vi "Ltree array to JSON.vi"(10 "Values":string[](array[string]), 11 "Names":string[][](array[string])) -> (3 "JSON String":string)   [LabVIEW 2019, in "Userlib.lvlib"]
uses:
  Userlib.lvlib
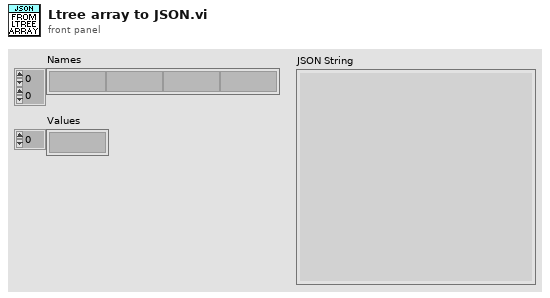
[diagram p1: front panel]
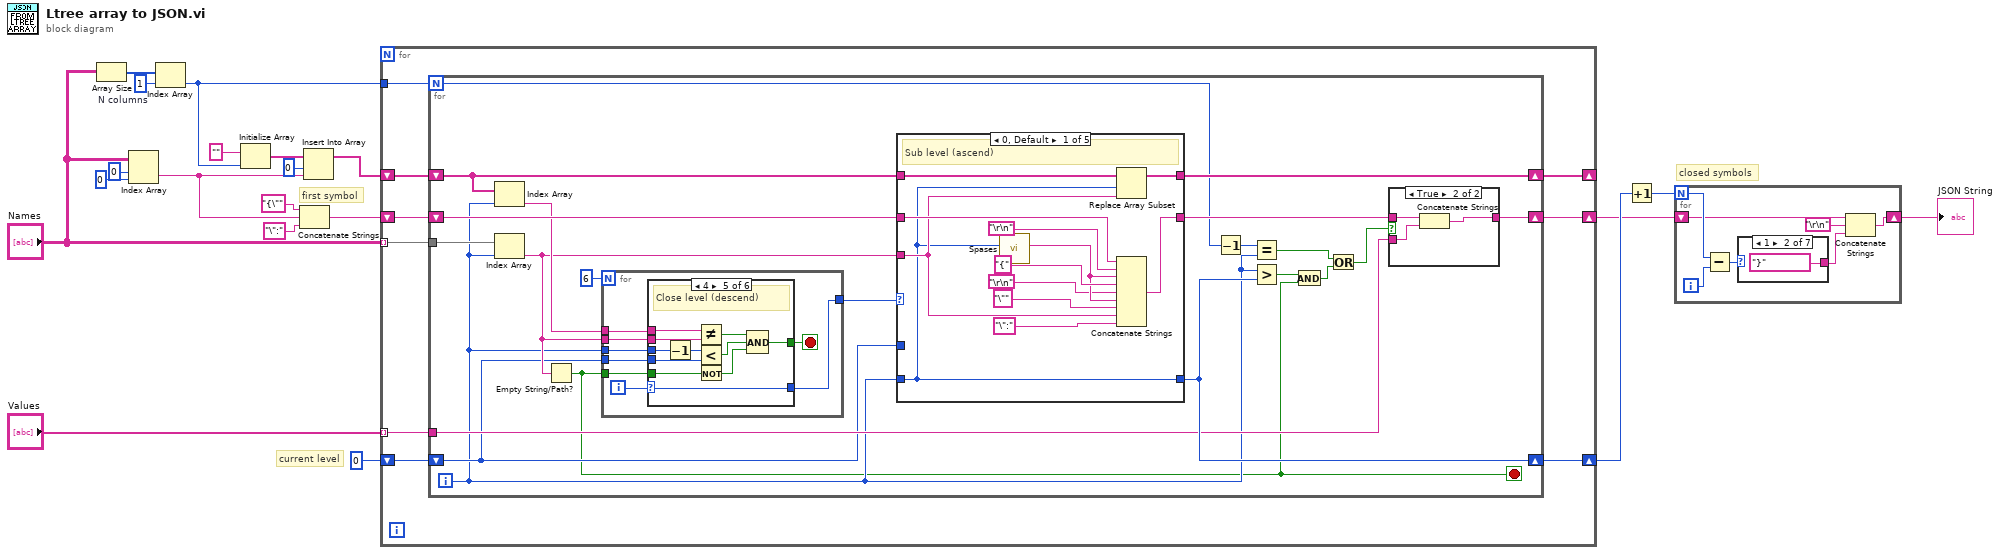
[diagram p0: block diagram]
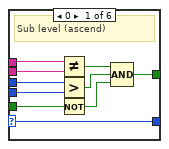
[diagram p2: hidden frame]
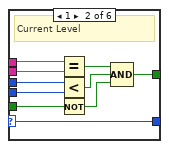
[diagram p3: hidden frame]
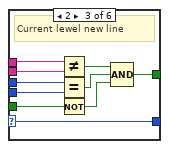
[diagram p4: hidden frame]
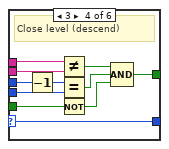
[diagram p5: hidden frame]
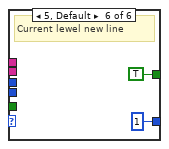
[diagram p6: hidden frame]
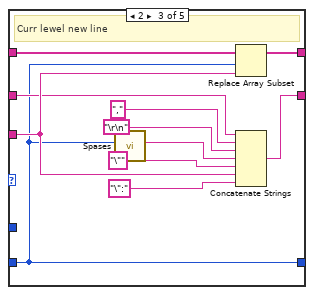
[diagram p8: hidden frame]
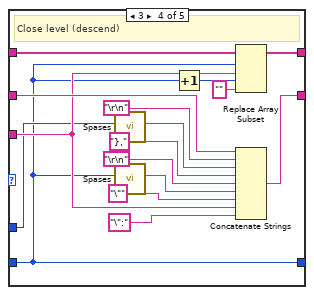
[diagram p9: hidden frame]
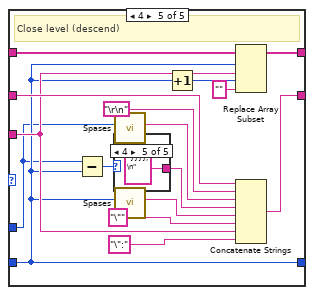
[diagram p10: hidden frame]
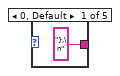
[diagram p11: hidden frame]
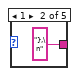
[diagram p12: hidden frame]
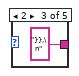
[diagram p13: hidden frame]
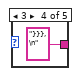
[diagram p14: hidden frame]
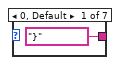
[diagram p16: hidden frame]
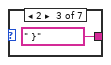
[diagram p17: hidden frame]
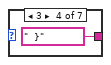
[diagram p18: hidden frame]
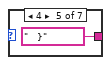
[diagram p19: hidden frame]
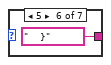
[diagram p20: hidden frame]
diagram:
  w18 = 1  # N columns
  # "closed symbols"
  # "first symbol"
  # "current level"
  n1 = Array Size(array="Names") -> (size(s)=w19:i32[])
  n2 = Index Array(array="Names", index (row)=0, index (col)=0 ("disabled index (col)")) -> (element=w10:string)
  n3 = Index Array(array=w19, index=w18) -> (element=w5:i32)
  n4 = Initialize Array("", w5) -> (w12:string[])
  n5 = Concatenate Strings("{\"", w10, "\":" ("string")) -> (w13:string)
  n6 = Insert Into Array(array=w12, index=0, new element=w10) -> (w9:string[])
  n7 = for {
    tunnel: "Names" -> [w26] mode=indexing
    shift-right: [w27] -> w7
    shift-left: w13 -> [w28]
    shift-right: [w24] -> w8
    shift-left: 0 -> [w25]
    shift-right: [w23] -> _
    shift-left: w9 -> [w29]
    tunnel: w5 -> [w22]
    tunnel: "Values" -> [w21] mode=indexing
    n8 = for {
      N: w22 -> [w34]
      tunnel: w26 -> [w47]
      shift-right: [w49] -> w23
      shift-left: w29 -> [w50]
      shift-right: [w45] -> w27
      shift-left: w28 -> [w48]
      shift-right: [w43] -> w24
      shift-left: w25 -> [w39]
      tunnel: w21 -> [w42]
      i -> [w35]
      stop <- w30 stop-if-true
      n9 = Index Array(array=w50, index=w35) -> (element=w41:string)
      n10 = Index Array(array=w47, index=w35) -> (element=w40:string)
      n11 = Empty String/Path?(string/path=w40) -> (empty?=w30:bool)
      n12 = for {
        N: 6 -> [_]
        tunnel: w41 -> [w58]
        tunnel: w40 -> [w57]
        tunnel: w39 -> [w56]
        tunnel: w30 -> [w55]
        tunnel: w35 -> [w54]
        tunnel: [w51] -> w38
        i -> [w52]
        stop <- w53 stop-if-true
        n13 = case shown="4" w52 {
          selector: w52 -> [w59 w69 w79 w89 w100 _]
          tunnel: w58 -> [w65 w75 w85 w96 w107 _]
          tunnel: w57 -> [w64 w74 w84 w95 w106 _]
          tunnel: w54 -> [w63 w73 w83 w91 w102 _]
          tunnel: w56 -> [w62 w72 w82 w94 w105 _]
          tunnel: w55 -> [w61 w71 w81 w93 w104 _]
          tunnel: [w60 w70 w80 w92 w103 TRUE] -> w53
          tunnel: [w59 w69 w79 w89 w100 1] -> w51
          frame 0 {
            # "Sub level (ascend)"
            n14 = Not Equal?(x=w65, y=w64) -> (x != y?=w68:bool)
            n15 = Greater?(x=w63, y=w62) -> (0:w67:bool)
            n16 = Not(x=w61) -> (.not. x?=w66:bool)
            n17 = Compound Arithmetic op=AND(w68, w67, w66) -> (w60:bool)
          }
          frame 1 {
            # "Current Level"
            n18 = Equal?(x=w75, y=w74) -> (x = y?=w78:bool)
            n19 = Less?(x=w73, y=w72) -> (x < y?=w77:bool)
            n20 = Not(x=w71) -> (.not. x?=w76:bool)
            n21 = Compound Arithmetic op=AND(w78, w77, w76) -> (w70:bool)
          }
          frame 2 {
            # "Current lewel new line"
            n22 = Not Equal?(x=w85, y=w84) -> (x != y?=w88:bool)
            n23 = Equal?(x=w83, y=w82) -> (x = y?=w87:bool)
            n24 = Not(x=w81) -> (.not. x?=w86:bool)
            n25 = Compound Arithmetic op=AND(w88, w87, w86) -> (w80:bool)
          }
          frame 3 {
            # "Close level (descend)"
            n26 = Decrement(x=w91) -> (x-1=w90:i32)
            n27 = Not Equal?(x=w96, y=w95) -> (x != y?=w99:bool)
            n28 = Equal?(x=w90, y=w94) -> (x = y?=w98:bool)
            n29 = Not(x=w93) -> (.not. x?=w97:bool)
            n30 = Compound Arithmetic op=AND(w99, w98, w97) -> (w92:bool)
          }
          frame 4 {
            # "Close level (descend)"
            n31 = Decrement(x=w102) -> (x-1=w101:i32)
            n32 = Not Equal?(x=w107, y=w106) -> (x != y?=w110:bool)
            n33 = Less?(x=w101, y=w105) -> (x < y?=w109:bool)
            n34 = Not(x=w104) -> (.not. x?=w108:bool)
            n35 = Compound Arithmetic op=AND(w110, w109, w108) -> (w103:bool)
          }
          frame 5, Default {
            # "Current lewel new line"
          }
        }
      }
      n36 = case shown="0, Default" w38 {
        tunnel: w40 -> [w119 _ w134 w148 w165]
        tunnel: [w124 w127 w138 w154 w170] -> w46
        tunnel: w50 -> [w123 w125 w137 w153 w169]
        tunnel: w35 -> [w115 _ w129 w141 w158]
        tunnel: [w122 w125 w136 w152 w168] -> w49
        tunnel: w48 -> [w121 w127 w131 w151 w167]
        tunnel: w39 -> [_ w126 _ w143 w156]
        tunnel: [w115 w126 w129 w141 w158] -> w43
        frame 0, Default {
          # "Sub level (ascend)"
          n37 = call "Spases.vi"("Numeric"=w115) -> ("spaces"=w114:string)  [unwired: 10 in]
          n38 = Replace Array Subset(array=w123, new element=w119, index=w115) -> (w122:string[])
          n39 = Concatenate Strings(w121, "\r\n", w114, "{", "\r\n", w114, "\"", w119, "\":" ("string")) -> (w124:string)
        }
        frame 1 {
          # "Current Level"
        }
        frame 2 {
          # "Curr lewel new line"
          n40 = call "Spases.vi"("Numeric"=w129) -> ("spaces"=w128:string)  [unwired: 10 in]
          n41 = Replace Array Subset(array=w137, new element=w134, index=w129) -> (w136:string[])
          n42 = Concatenate Strings(w131, ",", "\r\n", w128, "\"", w134, "\":" ("string")) -> (w138:string)
        }
        frame 3 {
          # "Close level (descend)"
          n43 = call "Spases.vi"("Numeric"=w143) -> ("spaces"=w142:string)  [unwired: 10 in]
          n44 = call "Spases.vi"("Numeric"=w141) -> ("spaces"=w140:string)  [unwired: 10 in]
          n45 = Increment(x=w141) -> (x+1=w145:i32)
          n46 = Replace Array Subset(array=w153, new element #1=w148, index #1=w141, new element #2="" ("new element/subarray"), index #2=w145) -> (w152:string[])
          n47 = Concatenate Strings(w151, "\r\n", w142, "},", "\r\n", w140, "\"", w148, "\":" ("string")) -> (w154:string)
        }
        frame 4 {
          # "Close level (descend)"
          n48 = Subtract(x=w156, y=w158) -> (x-y=w162:i32)
          n49 = case shown="4" w162 {
            tunnel: ["},\n" "},\n" "}},\n" "}}},\n" "}}}},\n"] -> w161
            frame 0, Default {
            }
            frame 1 {
            }
            frame 2 {
            }
            frame 3 {
            }
            frame 4 {
            }
          }
          n50 = call "Spases.vi"("Numeric"=w156) -> ("spaces"=w155:string)  [unwired: 10 in]
          n51 = call "Spases.vi"("Numeric"=w158) -> ("spaces"=w157:string)  [unwired: 10 in]
          n52 = Increment(x=w158) -> (x+1=w160:i32)
          n53 = Replace Array Subset(array=w169, new element #1=w165, index #1=w158, new element #2="" ("new element/subarray"), index #2=w160) -> (w168:string[])
          n54 = Concatenate Strings(w167, "\r\n", w155, w161, w157, "\"", w165, "\":" ("string")) -> (w170:string)
        }
      }
      n55 = Decrement(x=w34) -> (x-1=w36:i32)
      n56 = Equal?(x=w36, y=w35) -> (x = y?=w32:bool)
      n57 = Greater?(x=w35, y=w43) -> (0:w31:bool)
      n58 = And(x=w31, y=w30) -> (x .and. y?=w44:bool)
      n59 = Or(x=w32, y=w44) -> (x .or. y?=w33:bool)
      n60 = case shown="True" w33 {
        tunnel: w46 -> [w176 w179]
        tunnel: [w176 w177] -> w45
        tunnel: w42 -> [_ w178]
        frame False {
        }
        frame True {
          n61 = Concatenate Strings(w179, w178) -> (w177:string)
        }
      }
    }
  }
  n62 = Increment(x=w8) -> (x+1=w4:i32)
  n63 = for {
    N: w4 -> [w186]
    shift-right: [w182] -> w1
    shift-left: w7 -> [w183]
    i -> [w185]
    n64 = Subtract(x=w186, y=w185) -> (x-y=w184:i32)
    n65 = case shown="1" w184 {
      tunnel: ["}" ("end") "}" ("end") " }" ("end") "  }" ("end") "   }" ("end") "    }" ("end") "     }" ("end")] -> w180
      frame 0, Default {
      }
      frame 1 {
      }
      frame 2 {
      }
      frame 3 {
      }
      frame 4 {
      }
      frame 5 {
      }
      frame 6 {
      }
    }
    n66 = Concatenate Strings(w183, "\r\n", w180) -> (w182:string)
  }
  "JSON String" <- w1
